vi "No User Defined Path found--error.vi"(11 "Additional Info":string) -> (0 "error out":errorcluster)   [LabVIEW 2022 SP3, in "hse-application.lvclass"]
doc: "No User Defined Path found with name %s\n\n____\nHAMPEL SOFTWARE ENGINEERING v3.8.0 (2023-12-18 14:41)"
uses:
  hse-application.lvclass
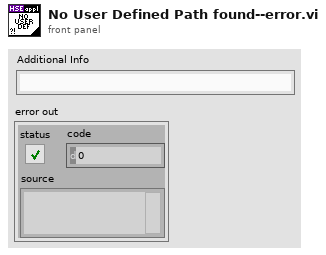
[diagram p1: front panel]
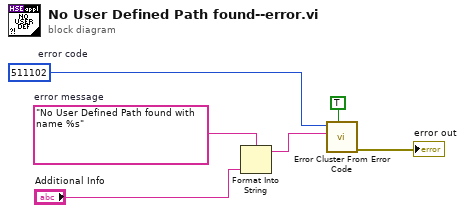
[diagram p0: block diagram]
diagram:
  w3 = "No User Defined Path found with name %s"  # error message
  w5 = 511102  # error code
  n1 = Format Into String(format string=w3, "Additional Info") -> (resulting string=w2:string)  [unwired: 2 in, 1 out]
  n2 = call <vilib>:"Error Cluster From Error Code.vi"("show call chain? (False)"=TRUE, "error message (\"\")"=w2, "error code (0)"=w5) -> ("error out"=→"error out":errorcluster)  [unwired: 6 in]
